vi "IMU Xform.vi"(10 "Pitch":dbl, 11 "Roll":dbl) -> (3 "Thigh Angle":dbl)   [LabVIEW 2018]
uses:
  <vilib>/Analysis/baseanly.llb/Real A x B.vi
  <vilib>/Analysis/NI_AALBase.lvlib
panel:
  out "Second output":dbl
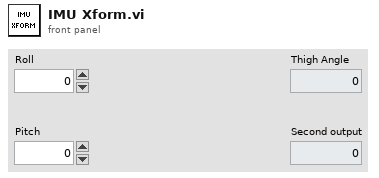
[diagram p1: front panel]
types:
  T1 = typedef "NI_Matrix.lvlib/RealMatrix.ctl" = dbl[][]
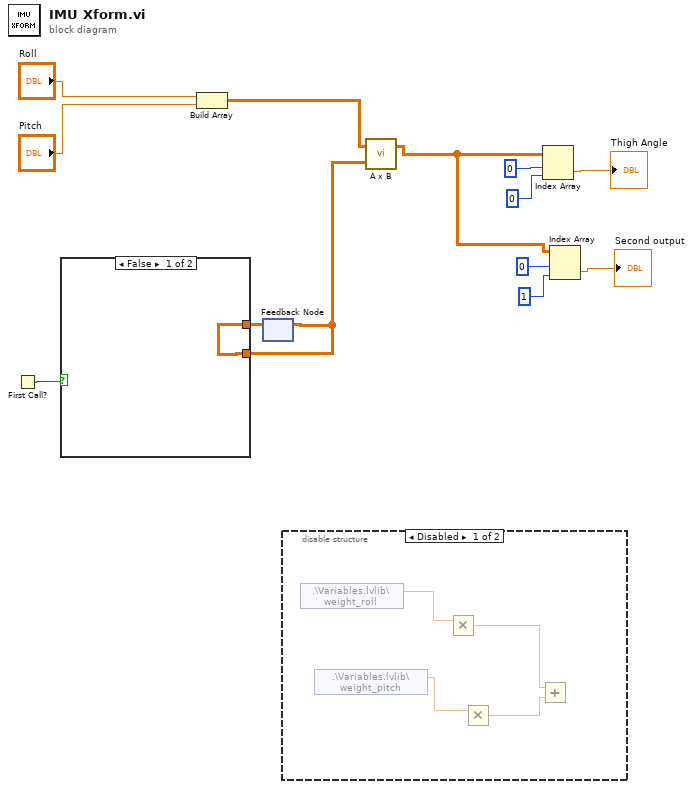
[diagram p0: block diagram]
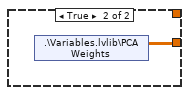
[diagram p2: hidden frame]
diagram:
  n1 = First Call?() -> (First Call?: T/F=w3:bool)
  n2 = Build Array("Roll", "Pitch") -> (w11:T1)
  n3 = feedback #1() -> (w1:dbl[][])  [unwired: 1 in]
  n4 = case shown="False" w3 {
    tunnel: [w14 w15] -> w2
    tunnel: w1 -> [w14 _]
    frame False {
    }
    frame True {
      n5 = shared-variable ".\\Variables.lvlib\\PCA Weights"() -> (w15:dbl[][])  [unwired: 1 in, 1 out]
    }
  }
  n6 = feedback-in #1(w2) -> ()
  n7 = disable-structure shown="Disabled" {
    frame Disabled {
      n8 = shared-variable ".\\Variables.lvlib\\weight_roll"() -> (w16:dbl)  [unwired: 1 in, 1 out]
      n9 = shared-variable ".\\Variables.lvlib\\weight_pitch"() -> (w17:dbl)  [unwired: 1 in, 1 out]
      n10 = Multiply(x=w16) -> (x*y=w19:dbl)  [unwired: 1 in]
      n11 = Multiply(x=w17) -> (x*y=w18:dbl)  [unwired: 1 in]
      n12 = Add(x=w19, y=w18) -> ()  [unwired: 1 out]
    }
    frame Enabled {
    }
  }
  n13 = call-poly <vilib>:"A x B.vi"("B"=w2, "A"=w11) -> ("A x B"=w6:T1)  [unwired: 1 out]
  n14 = Index Array(array=w6, index (row)=0, index (col)=0) -> (element=→"Thigh Angle":dbl)
  n15 = Index Array(array=w6, index (row)=0, index (col)=1) -> (element=→"Second output":dbl)
